vi "Configure Delay Trigger.vi"(0 "VISA resource name":refnum<visa-resource-name>, 1 "Trigger Slope (0: Rising)":u16(ring) items=["Rising", "Falling"], 2 "Trigger Coupling (0 : DC)":u16(ring) items=["DC", "HF Reject", "LF Reject", "Noise Reject"], 5 "Enable Delay Trigger (T: Enable)":bool=TRUE, 7 "Trigger Source (0: Channel 1)":u16(ring) items=["Channel 1", "Channel 2", "Channel 3", "Channel 4", "RF", "AC Line", "Aux"], 9 "Trigger Level (0.0 V)":dbl, 11 "error in (no error)":errorcluster, 12 "B Trigger After A":T1={"Trigger Mode (0: Trigger After Time) "=0, "Time (4.0ns)"=4e-09, "Events (1)"=1} {"Trigger Mode (0: Trigger After Time)" items=["Trigger After Time", "Trigger After Events"]}) -> (4 "VISA resource name out":refnum<visa-resource-name>, 15 "error out":errorcluster)   [LabVIEW 2016, in "Tektronix DPO MSO 2000 4000 Series.lvlib"]
doc: "Configures delay edge trigger settings. A delay edge trigger occurs after the main edge trigger event, when the trigger signal passes through the voltage threshold that you specify and has the slope that you specify.\n\nThe delay trigger is effective only when you set the edge trigger as the main trigger.\n\n<B>Note:</B>\n\nThis VI is not valid for DPO2K And MSO2K series."
uses:
  Tektronix DPO MSO 2000 4000 Series.lvlib
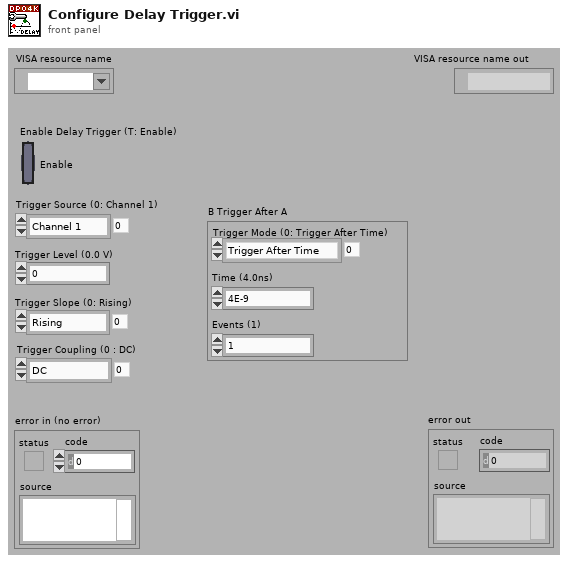
[diagram p1: front panel]
types:
  T1 = cluster{"Trigger Mode (0: Trigger After Time) ":u16, "Time (4.0ns)":dbl, "Events (1)":i32}
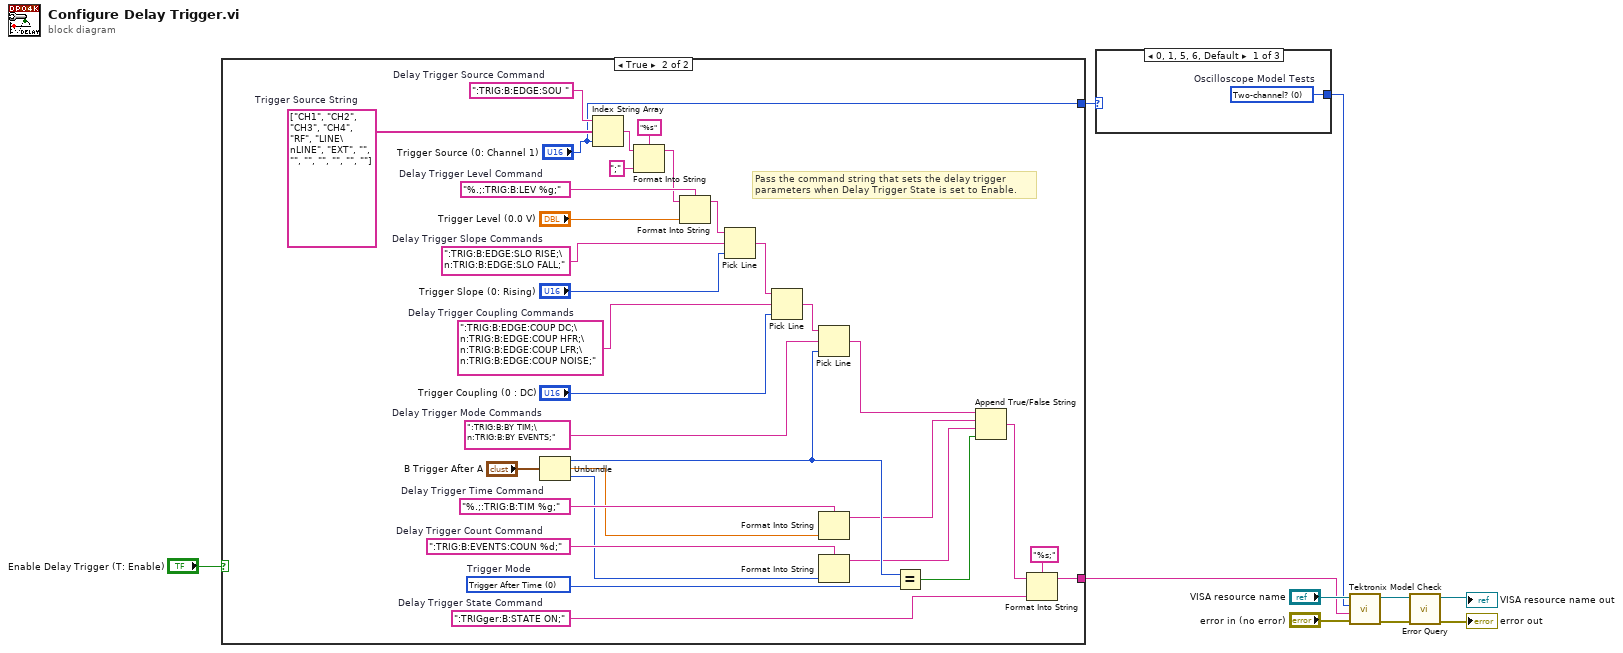
[diagram p0: block diagram]
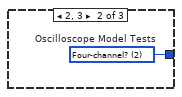
[diagram p2: hidden frame]
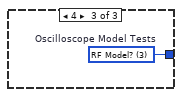
[diagram p3: hidden frame]
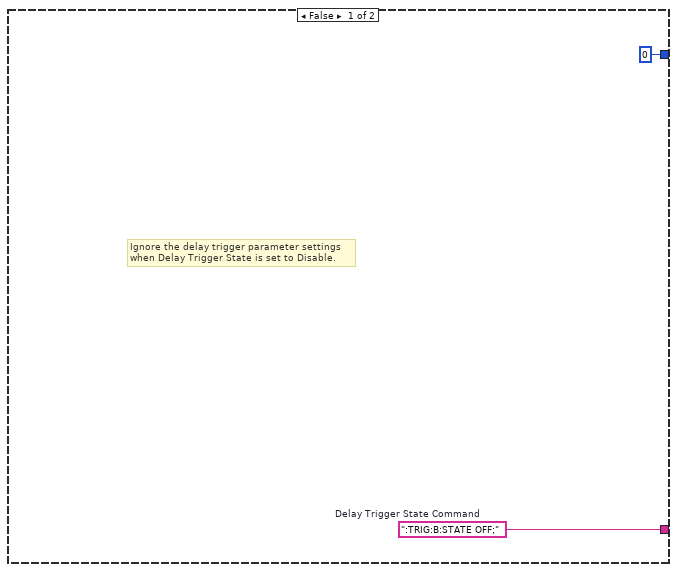
[diagram p4: hidden frame]
diagram:
  n1 = case shown="True" "Enable Delay Trigger (T: Enable)" {
    tunnel: [w12 w14] -> w5
    tunnel: [u16 0 ("Trigger Source (0: Channel 1)") "Trigger Source (0: Channel 1)"] -> w2
    frame False {
      w12 = ":TRIG:B:STATE OFF;"  # Delay Trigger State Command
      # "Ignore the delay trigger parameter settings  \nwhen Delay Trigger State is set to Disable."
    }
    frame True {
      w25 = ":TRIG:B:EVENTS:COUN %d;"  # Delay Trigger Count Command
      w27 = "%.;:TRIG:B:TIM %g;"  # Delay Trigger Time Command
      w29 = ":TRIG:B:BY TIM;\n:TRIG:B:BY EVENTS;"  # Delay Trigger Mode Commands
      w22 = u16 0 items=["Trigger After Time", "Trigger After Events"]  # Trigger Mode
      w33 = ":TRIG:B:EDGE:COUP DC;\n:TRIG:B:EDGE:COUP HFR;\n:TRIG:B:EDGE:COUP LFR;\n:TRIG:B:EDGE:COUP NOISE;"  # Delay Trigger Coupling Commands
      w35 = ":TRIG:B:EDGE:SLO RISE;\n:TRIG:B:EDGE:SLO FALL;"  # Delay Trigger Slope Commands
      w39 = "%.;:TRIG:B:LEV %g;"  # Delay Trigger Level Command
      w43 = ":TRIG:B:EDGE:SOU "  # Delay Trigger Source Command
      w17 = ":TRIGger:B:STATE ON;"  # Delay Trigger State Command
      w44 = string[] ["CH1", "CH2", "CH3", "CH4", "RF", "LINE\nLINE", "EXT", "", "", "", "", "", "", ""]  # Trigger Source String
      # "Pass the command string that sets the delay trigger\nparameters when Delay Trigger State is set to Enable."
      n2 = Unbundle("B Trigger After A") -> ("Trigger Mode (0: Trigger After Time)"=w23:u16, "Time (4.0ns)"=w26:dbl, "Events (1)"=w24:i32)
      n3 = Index String Array(1:"Trigger Source (0: Channel 1)", 2:w44, 3:w43) -> (0:w41:string)
      n4 = Format Into String(format string="%s", initial string=w41, ";" ("input 1")) -> (resulting string=w38:string)  [unwired: 1 in, 1 out]
      n5 = Format Into String(format string=w39, initial string=w38, "Trigger Level (0.0 V)") -> (resulting string=w36:string)  [unwired: 1 in, 1 out]
      n6 = Pick Line(string ("")=w36, multi-line string=w35, line index="Trigger Slope (0: Rising)") -> (output string=w32:string)
      n7 = Pick Line(string ("")=w32, multi-line string=w33, line index="Trigger Coupling (0 : DC)") -> (output string=w28:string)
      n8 = Pick Line(string ("")=w28, multi-line string=w29, line index=w23) -> (output string=w20:string)
      n9 = Format Into String(format string=w27, w26) -> (resulting string=w19:string)  [unwired: 2 in, 1 out]
      n10 = Format Into String(format string=w25, w24) -> (resulting string=w18:string)  [unwired: 2 in, 1 out]
      n11 = Equal?(x=w23, y=w22) -> (x = y?=w21:bool)
      n12 = Append True/False String(1:w21, 2:w18, 3:w19, 4:w20) -> (0:w16:string)
      n13 = Format Into String(format string="%s;", initial string=w16, w17) -> (resulting string=w14:string)  [unwired: 1 in, 1 out]
    }
  }
  n14 = case shown="0, 1, 5, 6, Default" w2 {
    tunnel: [w45 w46 w47] -> w1
    frame 0, 1, 5, 6, Default {
      w45 = u16 0 items=["Two-channel?", "Digital Model?", "Four-channel?", "RF Model?"]  # Oscilloscope Model Tests
    }
    frame 2, 3 {
      w46 = u16 2 items=["Two-channel?", "Digital Model?", "Four-channel?", "RF Model?"]  # Oscilloscope Model Tests
    }
    frame 4 {
      w47 = u16 3 items=["Two-channel?", "Digital Model?", "Four-channel?", "RF Model?"]  # Oscilloscope Model Tests
    }
  }
  n15 = call "Tektronix Model Check.vi"("error in (no error)"="error in (no error)", "Command String"=w5, "Oscilloscope Model Tests (3: RF Model?)"=w1, "VISA resource name"="VISA resource name") -> ("error out"=w3:errorcluster, "VISA resource name out"=w4:refnum<visa-resource-name>)  [unwired: 6 in]
  n16 = call "Error Query.vi"("error in (no error)"=w3, "VISA resource name"=w4) -> ("error out"=→"error out":errorcluster, "VISA resource name out"=→"VISA resource name out":refnum<visa-resource-name>)  [unwired: 6 in, 2 out]
